vi "Cycle Complete.vi"(8 "error in (no error)":errorcluster, 11 "Active in":refnum<class "Active.lvclass">) -> (0 "error out":errorcluster, 3 "State Actor out":refnum<class "State Actor.lvclass">)   [LabVIEW 2024, in "Sample State Actor.lvlib" / "Active.lvclass"]
uses:
  State Actor/State Actor.lvclass
  Active.lvclass
  Active.lvclass/Active.ctl
  Idle/Idle.lvclass
  C:/Users/uspoaotto/Downloads/State Actor/Sample State Actor/Main/Main.lvclass
  C:/Users/uspoaotto/Downloads/State Actor/State Actor/State Actor.lvclass
  C:/Program Files (x86)/National Instruments/LabVIEW 2024/vi.lib/ActorFramework/Actor/Actor.lvclass
  C:/Users/uspoaotto/Downloads/State Actor/Sample State Actor/Idle/Idle.lvclass
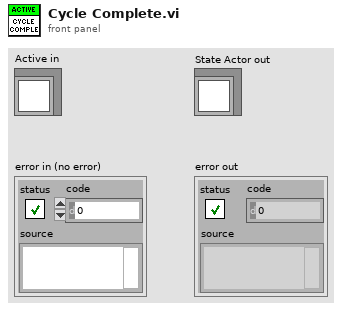
[diagram p1: front panel]
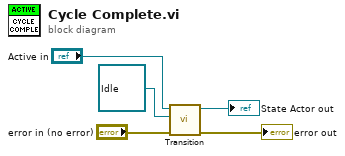
[diagram p0: block diagram]
diagram:
  n1 = call-dynamic "Transition.vi"("error in (no error)"="error in (no error)", "Target State Actor in"=refnum<class "Idle.lvclass"> refnum ("Sample State Actor.lvlib:Idle.lvclass"), "State Actor in"="Active in") -> ("error out"=→"error out":errorcluster, "State Actor out"=→"State Actor out":refnum<class "State Actor.lvclass">)  [unwired: 7 in]
